vi "Test-SMObase.vi"() -> ()   [LabVIEW 2013]
uses:
  src/SMO/Typedefs/SMOState --Enum.ctl
  src/SMO/SMO.lvclass
  src/Registry/Registry-SMO.lvclass
panel:
  out "Second Pump Qualified Name":string
  out "Registered":string[](array[string])
  out "First Pump Qualified Name":string
  out "Second Pump Instance Name":string
  out "First Pump Instance Name":string
  out "Warning 42 expected":errorcluster
  out "System Name":string
  out "SMO State":T1
  in  "Stop":bool
  out "error out":errorcluster
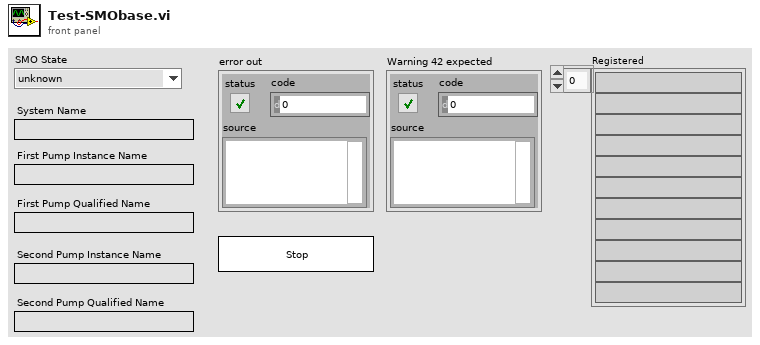
[diagram p1: front panel]
types:
  T1 = typedef "SMO.lvclass/SMOState --Enum.ctl" = enum16{"unknown", "Created", "Started", "Stopped"}
  T2 = typedef "Registry-SMO.lvclass/PublicRegistryEvents--Cluster.ctl" = cluster{"Register Event":refnum<user-event>, "Unregister Event":refnum<user-event>}
  T3 = typedef "SMO.lvclass/Public Events.ctl" = cluster{"Error":refnum<user-event>, "State":refnum<user-event>, "Reserve State":refnum<user-event>}
  T4 = cluster{"Event Registration Refnum":refnum<event-registration>}
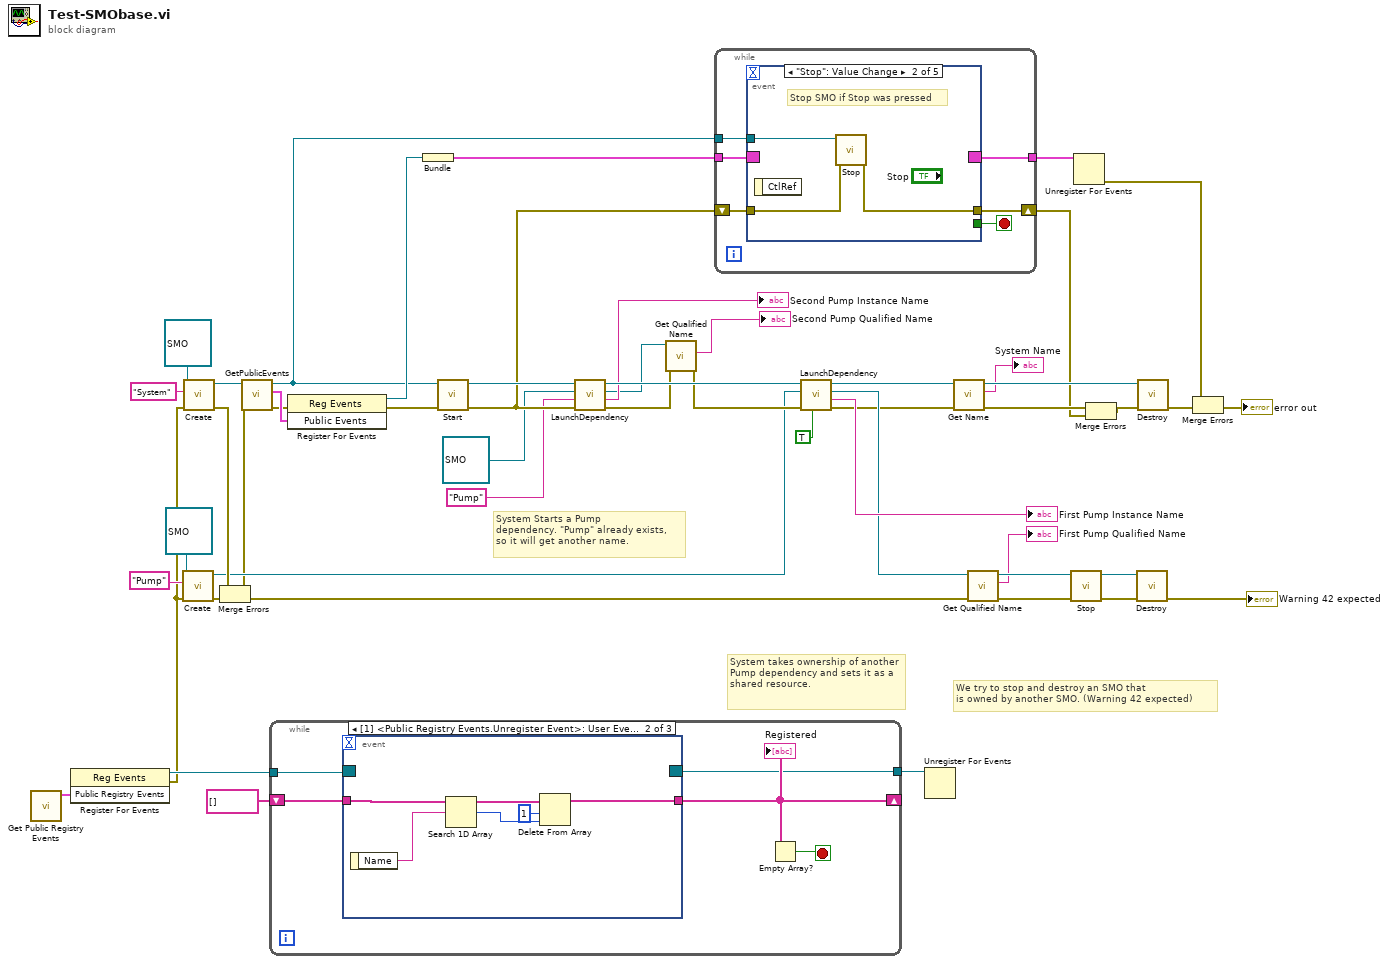
[diagram p0: block diagram]
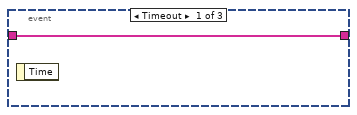
[diagram p2: hidden frame]
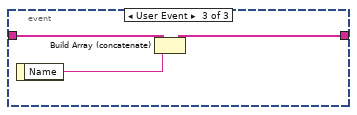
[diagram p3: hidden frame]
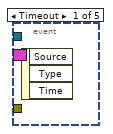
[diagram p4: hidden frame]
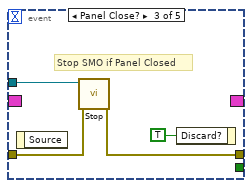
[diagram p5: hidden frame]
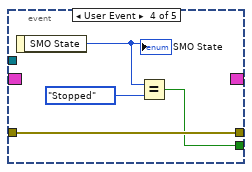
[diagram p6: hidden frame]
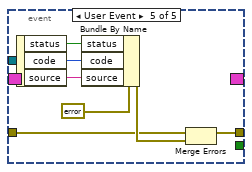
[diagram p7: hidden frame]
diagram:
  # "System Starts a Pump\ndependency. \"Pump\" already exists,\nso it will get another name."
  # "We try to stop and destroy an SMO that\nis owned by another SMO. (Warning 42 expected)"
  # "System takes ownership of another Pump dependency and sets it as a shared resource."
  n1 = call "Get Public Registry Events.vi"() -> ("Public Registry Events"=w16:T2)  [unwired: 10 in, 1 out]
  n2 = register-events(w16) -> (reference out=w15:refnum<event-registration>, error out=w14:errorcluster)  [unwired: 2 in]
  n3 = call "Create.vi"("error in (no error)"=w14, "Subsystem Name (optional)"="Pump", "SMO"=refnum<class "SMO.lvclass"> refnum ("SMO.lvclass")) -> ("error out"=w21:errorcluster, "SMO out"=w8:refnum<class "SMO.lvclass">)  [unwired: 6 in, 1 out]
  n4 = call "Create.vi"("error in (no error)"=w14, "Subsystem Name (optional)"="System", "SMO"=refnum<class "SMO.lvclass"> refnum ("SMO.lvclass")) -> ("error out"=w20:errorcluster, "SMO out"=w43:refnum<class "SMO.lvclass">)  [unwired: 6 in, 1 out]
  n5 = Merge Errors(w20, w21) -> (w4:errorcluster)
  n6 = call "GetPublicEvents.vi"("error in (no error)"=w4, "SMO"=w43) -> ("error out"=w40:errorcluster, "Public Events"=w42:T3, "SMO out"=w41:refnum<class "SMO.lvclass">)  [unwired: 7 in]
  n7 = while {
    tunnel: w15 -> [w55]
    shift-right: [w53] -> _
    shift-left: string[] [] -> [w54]
    tunnel: [w51] -> w12
    stop <- w52 stop-if-true
    n8 = event shown="[1] <Public Registry Events.Unregister Event>: User Event" {
      selector: w55 -> [_ _ _]
      dyn-events: [_ _ _] -> w51
      timeout: _ -> [_ _ _]
      tunnel: w54 -> [w56 w60 w64]
      tunnel: [w56 w59 w62] -> w53
      event Timeout {
        n9 = event-data() -> ()  [unwired: 1 in, 1 out]
      }
      event User Event {
        n10 = event-data() -> ("Name"=w61:string)  [unwired: 1 in]
        n11 = Search 1D Array(1D array=w60, element=w61) -> (index of element=w58:i32)  [unwired: 1 in]
        n12 = Delete From Array(array=w60, length=1, index=w58) -> (array with subset deleted=w59:string[])  [unwired: 1 out]
      }
      event User Event {
        n13 = event-data() -> ("Name"=w63:string)  [unwired: 1 in]
        n14 = Build Array (concatenate)(w64, w63) -> (w62:string[])
      }
    }
    "Registered" <- w53
    n15 = Empty Array?(array=w53) -> (empty?=w52:bool)
  }
  n16 = register-events(error in=w40, w42) -> (reference out=w45:refnum<event-registration>, error out=w44:errorcluster)  [unwired: 1 in]
  n17 = Bundle("Event Registration Refnum"=w45) -> (w49:T4)  [unwired: 1 in]
  n18 = call "Start.vi"("error in (no error)"=w44, "SMO"=w41) -> ("error out"=w25:errorcluster, "SMO out"=w27:refnum<class "SMO.lvclass">)  [unwired: 8 in]
  n19 = call "LaunchDependency.vi"("error in (no error)"=w25, "Dependency Name"="Pump" ("Subsystem Name (optional)"), "Dependency Type"=refnum<class "SMO.lvclass"> refnum ("SMO.lvclass"), "SMO in"=w27) -> ("error out"=w10:errorcluster, "Unique Name"=→"Second Pump Instance Name":string, "Dependency Reference"=w11:refnum<class "SMO.lvclass">, "SMO out"=w26:refnum<class "SMO.lvclass">)  [unwired: 4 in]
  n20 = call "Get Qualified Name.vi"("error in (no error)"=w10, "SMO"=w11) -> ("error out"=w9:errorcluster, "Qualified Name"=→"Second Pump Qualified Name":string)  [unwired: 7 in, 1 out]
  n21 = while {
    shift-right: [w69] -> w1
    shift-left: w25 -> [w68]
    tunnel: w49 -> [w67]
    tunnel: [w66] -> w50
    tunnel: w41 -> [w65]
    stop <- w70 stop-if-true
    n22 = event shown="[1] \"Stop\": Value Change" {
      selector: w67 -> [_ _ _ _ _]
      dyn-events: [_ _ _ _ _] -> w66
      timeout: _ -> [_ _ _ _ _]
      tunnel: [_ _ _ w78 _] -> w70
      tunnel: w65 -> [_ w73 w77 _ _]
      tunnel: [_ w72 w76 w79 w82] -> w69
      tunnel: w68 -> [_ w71 w75 w79 w83]
      event Timeout {
        n23 = event-data() -> ()  [unwired: 1 in, 3 out]
      }
      event "Stop": Value Change {
        # "Stop SMO if Stop was pressed"
        n24 = event-data() -> ()  [unwired: 1 in, 1 out]
        n25 = call "Stop.vi"("error in (no error)"=w71, "SMO"=w73) -> ("error out"=w72:errorcluster)  [unwired: 8 in, 1 out]
      }
      event Panel Close? {
        # "Stop SMO if Panel Closed"
        n26 = event-data() -> ()  [unwired: 1 in, 1 out]
        n27 = call "Stop.vi"("error in (no error)"=w75, "SMO"=w77) -> ("error out"=w76:errorcluster)  [unwired: 8 in, 1 out]
        n28 = event-data("Discard?"=TRUE ("OK")) -> ()  [unwired: 1 in, 1 out]
      }
      event User Event {
        n29 = event-data() -> ("SMO State"=w81:T1)  [unwired: 1 in]
        "SMO State" <- w81
        n30 = Equal?(x=w81, y=SMOState_--Enum."Stopped") -> (x = y?=w78:bool)
      }
      event User Event {
        n31 = event-data() -> ("status"=w88:bool, "code"=w86:i32, "source"=w85:string)  [unwired: 1 in]
        n32 = Bundle By Name(cluster=errorcluster {"status"=FALSE, "code"=0, "source"=""} ("error constant"), "status"=w88, "code"=w86, "source"=w85) -> (w84:errorcluster)
        n33 = Merge Errors(w83, w84) -> (w82:errorcluster)
      }
    }
  }
  n34 = call "LaunchDependency.vi"("Shared Resource"=TRUE, "error in (no error)"=w9, "Dependency Type"=w8, "SMO in"=w26) -> ("error out"=w5:errorcluster, "Unique Name"=→"First Pump Instance Name":string, "Dependency Reference"=w7:refnum<class "SMO.lvclass">, "SMO out"=w6:refnum<class "SMO.lvclass">)  [unwired: 4 in]
  n35 = Unregister For Events(event registration refnum=w12) -> ()  [unwired: 1 in, 1 out]
  n36 = call "Get Name.vi"("error in (no error)"=w5, "SMO"=w6) -> ("error out"=w2:errorcluster, "Name"=→"System Name":string, "SMO out"=w38:refnum<class "SMO.lvclass">)  [unwired: 7 in]
  n37 = call "Get Qualified Name.vi"("error in (no error)"=w4, "SMO"=w7) -> ("error out"=w18:errorcluster, "Qualified Name"=→"First Pump Qualified Name":string, "SMO out"=w19:refnum<class "SMO.lvclass">)  [unwired: 7 in]
  n38 = call "Stop.vi"("error in (no error)"=w18, "SMO"=w19) -> ("error out"=w33:errorcluster, "SMO out"=w34:refnum<class "SMO.lvclass">)  [unwired: 8 in]
  n39 = Unregister For Events(event registration refnum=w50) -> (error out=w48:errorcluster)  [unwired: 1 in]
  n40 = Merge Errors(w2, w1) -> (w39:errorcluster)
  n41 = call "Destroy.vi"("error in (no error)"=w33, "SMO"=w34) -> ("error out"=→"Warning 42 expected":errorcluster)  [unwired: 9 in]
  n42 = call "Destroy.vi"("error in (no error)"=w39, "SMO"=w38) -> ("error out"=w46:errorcluster)  [unwired: 9 in]
  n43 = Merge Errors(w48, w46) -> (→"error out":errorcluster)
